vi "dt to f.vi"(11 "Period":i64) -> (3 "Frequency":dbl)   [LabVIEW 2021]
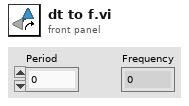
[diagram p1: front panel]
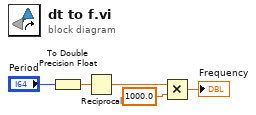
[diagram p0: block diagram]
diagram:
  n1 = To Double Precision Float(number="Period") -> (double precision float=w2:dbl)
  n2 = Reciprocal(x=w2) -> (1/x=w3:dbl)
  n3 = Multiply(x=w3, y=1000.0) -> (x*y=→"Frequency":dbl)
